vi "Init.vi"(8 "error in (no error)":errorcluster, 9 "vi reference":refnum<vi>, 10 "Graph_refs":T1, 11 "SettingsFile in":refnum<class "SettingsFile.lvclass">) -> (0 "error out":errorcluster, 2 "Save event":T3, 3 "SettingsFile out":refnum<class "SettingsFile.lvclass">)   [LabVIEW 2018, in "SettingsFile.lvclass"]
uses:
  SettingsFile.lvclass
  INI Save Event.ctl
  Save event.ctl
  Scope/controls/Graph_references.ctl
  Scope/controls/graph_controls.ctl
  SettingsFile.lvclass/SettingsFile.ctl
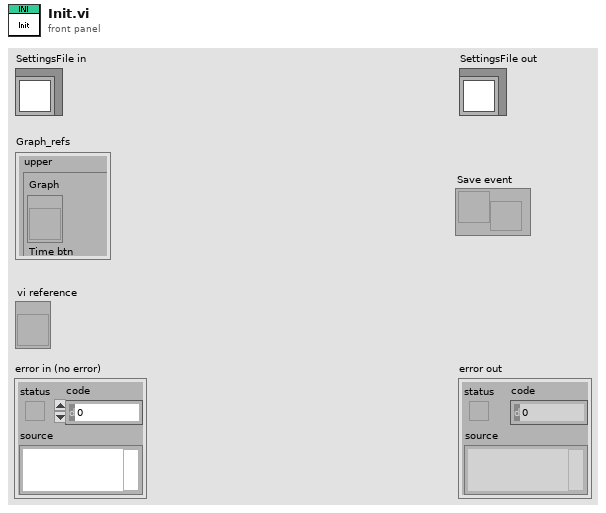
[diagram p1: front panel]
types:
  T1 = typedef "Graph_references.ctl" = cluster{"upper":T2, "lower":T2, "Freq graph":refnum<vi>, "Adaptive FF graph":refnum<vi>}
  T2 = typedef "graph_controls.ctl" = cluster{"Graph":refnum<vi>, "Time btn":refnum<vi>, "Amplitude btn":refnum<vi>, "Chart":refnum<vi>}
  T3 = typedef "INI Save Event.ctl" = refnum<user-event>
  T4 = typedef "Save event.ctl" = cluster{"Automatic":bool, "Save":bool}
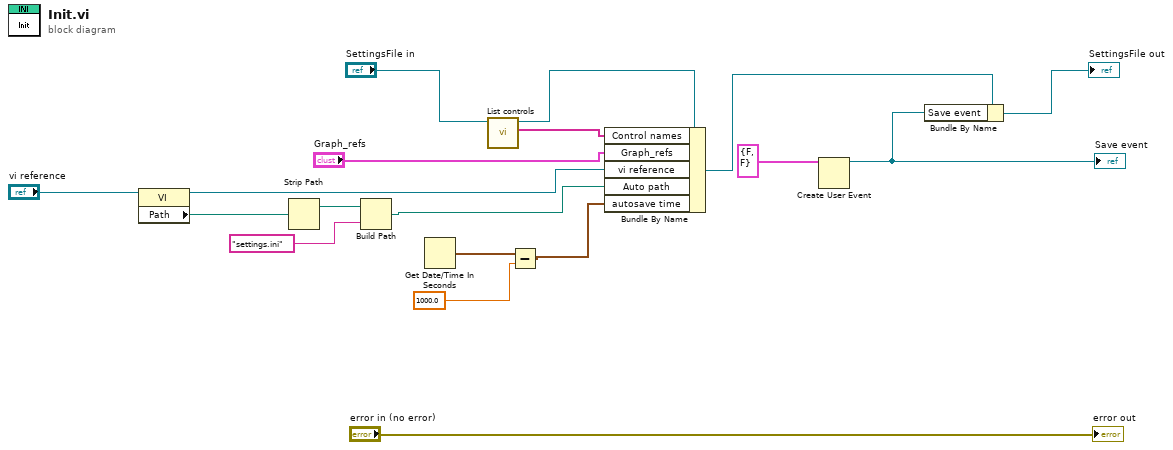
[diagram p0: block diagram]
diagram:
  n1 = property class="VI"(reference="vi reference") -> (reference out=w10:refnum<vi>, "Path"=w13:path)  [unwired: 1 in, 1 out]
  n2 = Strip Path(path=w13) -> (stripped path=w12:path)  [unwired: 1 out]
  n3 = Build Path(base path=w12, name or relative path="settings.ini") -> (appended path=w8:path)
  n4 = Get Date/Time In Seconds() -> (seconds since 1Jan1904=w7:timestamp)
  n5 = call-dynamic "List controls.vi"("SettingsFile in"="SettingsFile in") -> ("Control names"=w15:string[], "SettingsFile out"=w3:refnum<class "SettingsFile.lvclass">)  [unwired: 8 in, 1 out]
  n6 = Subtract(x=w7, y=1000.0) -> (x-y=w5:timestamp)
  n7 = Bundle By Name(cluster=w3, "Control names"=w15, "Graph_refs"="Graph_refs", "vi reference"=w10, "Auto path"=w8, "autosave time"=w5) -> (w1:refnum<class "SettingsFile.lvclass">)
  n8 = Create User Event(user event datatype=T4 {"Automatic"=FALSE, "Save"=FALSE} ("INI event")) -> (user event=w4:refnum<user-event>)  [unwired: 1 in, 1 out]
  "Save event" <- w4
  n9 = Bundle By Name(cluster=w1, "Save event"=w4) -> (→"SettingsFile out":refnum<class "SettingsFile.lvclass">)
  "error out" <- "error in (no error)"
